vi "GetNodeAccessMode.vi"(0 "nInputHandle":u64, 1 "strName":string, 2 "error in (no error)":errorcluster) -> (3 "nOuputHandle":u64, 4 "pemAccessMode":i32, 5 "GX_STATUS":i32, 6 "error out":errorcluster)   [LabVIEW 2016, in "GxLVLib.lvlib"]
uses:
  GxLVLib.lvlib
  GxIAPI.dll
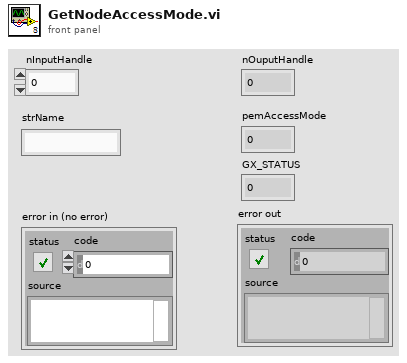
[diagram p1: front panel]
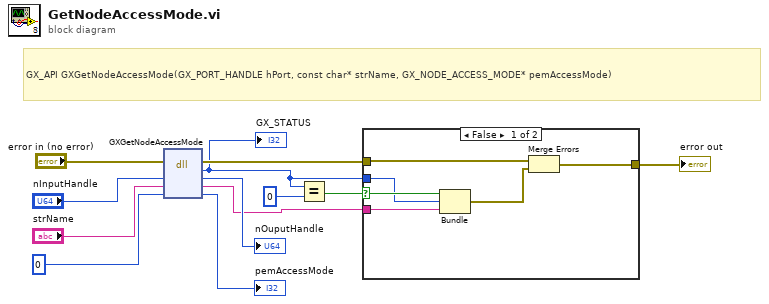
[diagram p0: block diagram]
diagram:
  # "GX_API GXGetNodeAccessMode(GX_PORT_HANDLE hPort, const char* strName, GX_NODE_ACCESS_MODE* pemAccessMode)"
  n1 = dll-call lib="GxIAPI.dll" fn="GXGetNodeAccessMode"(error in="error in (no error)", "hPort"="nInputHandle", "strName"="strName", "pemAccessMode"=0) -> (error out=w6:errorcluster, "GX_STATUS"=w2:i32, "hPort"=→"nOuputHandle":i64, "strName"=w3:string, "pemAccessMode"=→"pemAccessMode":i32)  [unwired: 2 in, 1 out]
  "GX_STATUS" <- w2
  n2 = Equal?(x=w2, y=0) -> (x = y?=w5:bool)
  n3 = case shown="False" w5 {
    selector: w5 -> [w15 _]
    tunnel: w6 -> [w18 w19]
    tunnel: [w17 w19] -> w7
    tunnel: w2 -> [w14 _]
    tunnel: w3 -> [w13 _]
    frame False {
      n4 = Bundle(w15, "GX_STATUS"=w14, "strName"=w13) -> (w16:cluster{bool, "GX_STATUS":i32, "strName":string})  [unwired: 1 in]
      n5 = Merge Errors(w18, w16) -> (w17:errorcluster)
    }
    frame True {
    }
  }
  "error out" <- w7
